vi "ap check new firmware version.vi"(10 "new_firmware_version":cluster{}, 11 "ap_handle":u32) -> (2 "function return":i32, 3 "ap_handle out":u32)   [LabVIEW 2019, in "apdm.lvlib"]
doc: "APDM_EXPORT int apdm_ap_check_new_firmware_version(apdm_ap_handle_t ap_handle, const int64_t new_firmware_version);"
uses:
  apdm.lvlib
  Lee Lab/CP FES Walking 2018/Code/Working/LabVIEW/apdm.dll
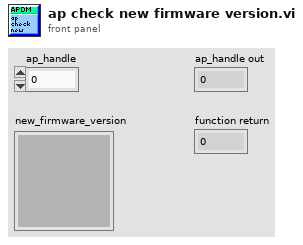
[diagram p1: front panel]
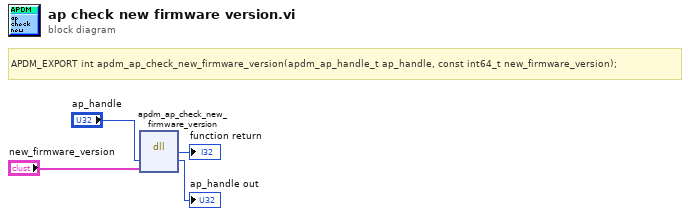
[diagram p0: block diagram]
diagram:
  # "APDM_EXPORT int apdm_ap_check_new_firmware_version(apdm_ap_handle_t ap_handle, const int64_t new_firmware_version);"
  n1 = dll-call lib="C:/Users/jfalesi/Dropbox/Lee Lab/CP FES Walking 2018/Code/Working/LabVIEW/apdm.*" fn="apdm_ap_check_new_firmware_version"("ap_handle"="ap_handle", "new_firmware_version"="new_firmware_version") -> (→"function return":i32, "ap_handle"=→"ap_handle out":u32)  [unwired: 4 in, 2 out]
